vi "CCE MGLD PMJD PF SubVI05.vi"(6 "Coordenadas":T2, 8 "DireccionMemoria":path, 9 "UMBRAL":u8(knob) scale=0.0..255.0, 10 "Tolerancia":dbl, 11 "Image":T1) -> (0 "Estado botella":string, 2 "Abolladuas?":bool)   [LabVIEW 2020]
uses:
  <vilib>/vision/Image Controls.llb/IMAQ Image.ctl
panel:
  out "Image 2":T1(plugin-control)
  out "Diferencia":dbl
  out "Memoria":picture
  out "Muestra":picture
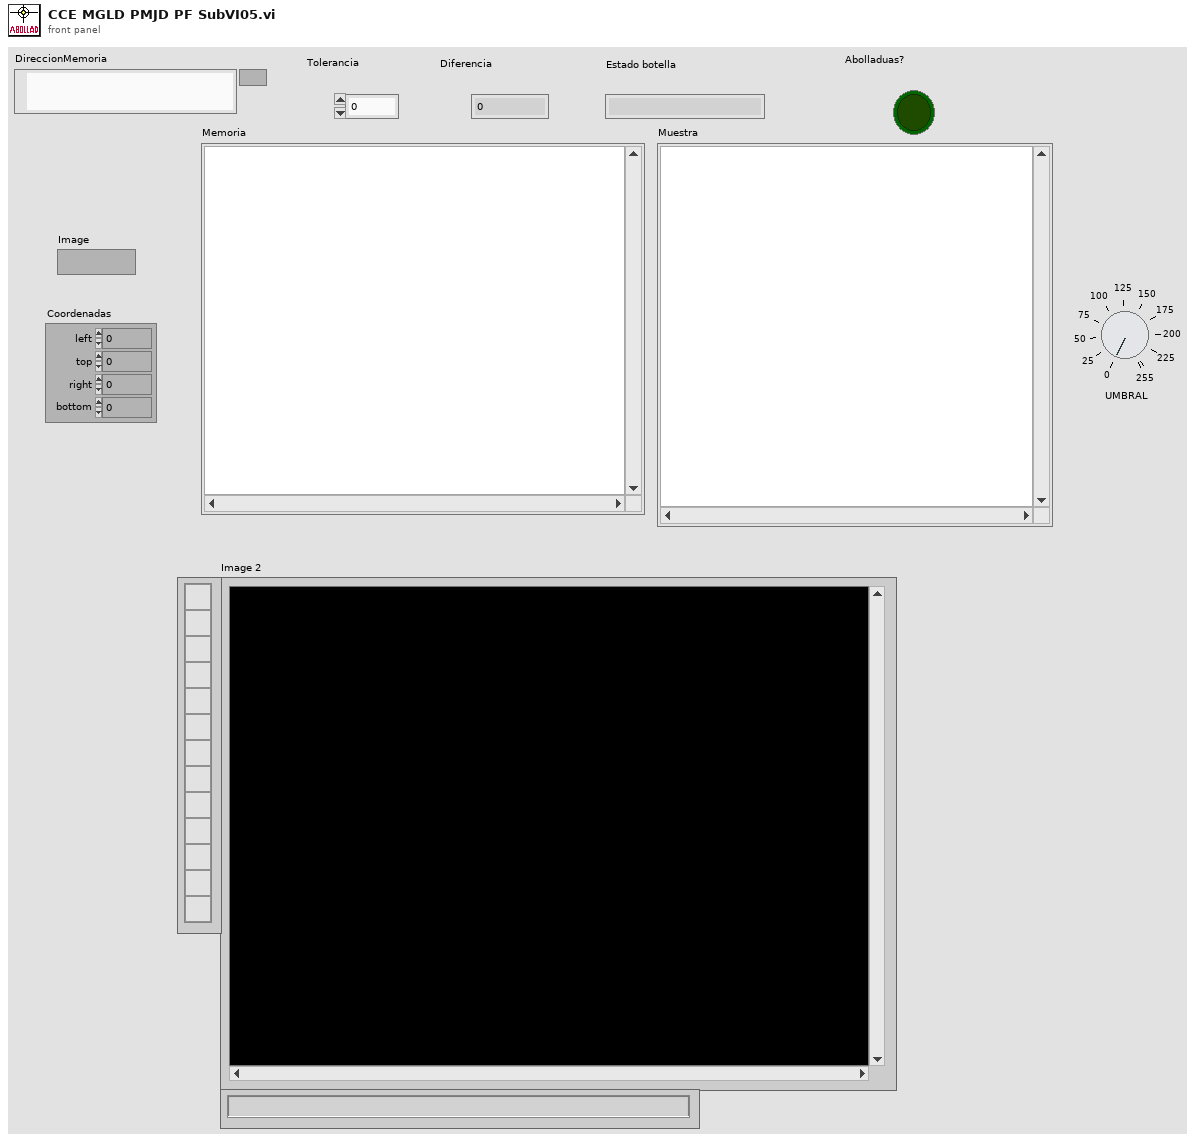
[diagram p1: front panel]
types:
  T1 = typedef "IMAQ Image.ctl" = refnum<image>
  T2 = cluster{"left":i16, "top":i16, "right":i16, "bottom":i16}
  T3 = typedef "Image Type" = u32
  T4 = typedef "imagedata.ctl" = cluster{"image type":i32, "image depth":i32, "image":u8[], "mask":u8[], "colors":u32[], "Rectangle":cluster{"left":i16, "top":i16, "right":i16, "bottom":i16}}
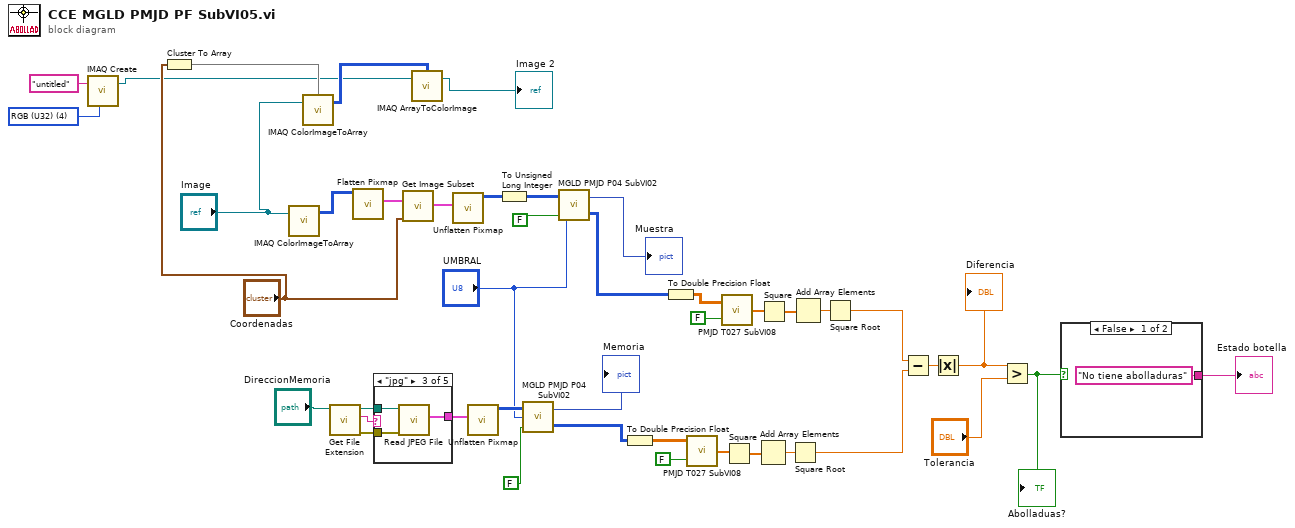
[diagram p0: block diagram]
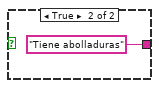
[diagram p2: hidden frame]
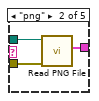
[diagram p4: hidden frame]
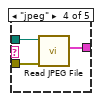
[diagram p5: hidden frame]
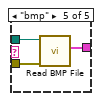
[diagram p6: hidden frame]
diagram:
  w1 = T3 4 items=["Grayscale (U8)", "Grayscale (I16)", "Grayscale (SGL)", "Complex (CSG)", "RGB (U32)", "HSL (U32)", "RGB (U64)", "Grayscale (U16)"] ("Image Type")
  n1 = call "IMAQ Create"("Image Name"="untitled", "Image Type"=w1) -> ("New Image"=w3:T1)  [unwired: 3 in, 1 out]
  n2 = Cluster To Array(cluster="Coordenadas") -> (array=w5:i16[])
  n3 = call "IMAQ ColorImageToArray"("Image"="Image") -> ("Image Pixels (U32)"=w10:u32[][])  [unwired: 3 in, 2 out]
  n4 = call "IMAQ ColorImageToArray"("Optional Rectangle"=w5, "Image"="Image") -> ("Image Pixels (U32)"=w7:u32[][])  [unwired: 2 in, 2 out]
  n5 = call <vilib>:"Get File Extension.vi"("file"="DireccionMemoria") -> ("error out"=w39:errorcluster, "lowercase file extension"=w41:string, "dup file"=w40:path)  [unwired: 6 in, 2 out]
  n6 = call <vilib>:"Flatten Pixmap.vi"("24-bit pixmap"=w10) -> ("image data"=w13:T4)  [unwired: 10 in]
  n7 = case shown="\"jpg\"" w41 {
    tunnel: w40 -> [_ w46 w47 w52 w54]
    tunnel: w39 -> [_ w45 w49 w51 w55]
    tunnel: [_ w44 w48 w50 w53] -> w38
    frame "False", Default {
    }
    frame "png" {
      n8 = call <vilib>:"Read PNG File.vi"("error in (no error)"=w45, "path to PNG file"=w46) -> ("image data"=w44:T4)  [unwired: 7 in, 2 out]
    }
    frame "jpg" {
      n9 = call <vilib>:"Read JPEG File.vi"("error in (no error)"=w49, "path to JPEG file"=w47) -> ("image data"=w48:T4)  [unwired: 7 in, 2 out]
    }
    frame "jpeg" {
      n10 = call <vilib>:"Read JPEG File.vi"("error in (no error)"=w51, "path to JPEG file"=w52) -> ("image data"=w50:T4)  [unwired: 7 in, 2 out]
    }
    frame "bmp" {
      n11 = call <vilib>:"Read BMP File.vi"("error in (no error)"=w55, "path to BMP file"=w54) -> ("image data"=w53:T4)  [unwired: 7 in, 2 out]
    }
  }
  n12 = call <vilib>:"Get Image Subset.vi"("subset rect"="Coordenadas", "image data"=w13) -> ("image subset"=w12:T4)  [unwired: 4 in, 1 out]
  n13 = call "IMAQ ArrayToColorImage"("Image Pixels (U32)"=w7, "Image"=w3) -> ("Image Out"=→"Image 2":T1)  [unwired: 3 in, 1 out]
  n14 = call <vilib>:"Unflatten Pixmap.vi"("image data"=w12) -> ("24-bit pixmap"=w11:u32[][])  [unwired: 4 in, 6 out]
  n15 = call <vilib>:"Unflatten Pixmap.vi"("image data"=w38) -> ("24-bit pixmap"=w36:u32[][])  [unwired: 4 in, 6 out]
  n16 = To Unsigned Long Integer(number=w11) -> (unsigned 32bit integer=w14:u32[][])
  n17 = call "MGLD PMJD P04 SubVI02.vi"("INVERTIDO?"=FALSE, "UMBRAL"="UMBRAL", "pixmap"=w36) -> ("Umbralizado"=w16:u8[][], "IMG"=→"Memoria":picture)
  n18 = call "MGLD PMJD P04 SubVI02.vi"("INVERTIDO?"=FALSE, "UMBRAL"="UMBRAL", "pixmap"=w14) -> ("Umbralizado"=w18:u8[][], "IMG"=→"Muestra":picture)
  n19 = To Double Precision Float(number=w16) -> (double precision float=w17:dbl[][])
  n20 = To Double Precision Float(number=w18) -> (double precision float=w19:dbl[][])
  n21 = call "PMJD T027 SubVI08.vi"("NORMALIZACIÓN"=FALSE, "f"=w17) -> ("MOMENTOS Hu"=w34:dbl[])
  n22 = call "PMJD T027 SubVI08.vi"("NORMALIZACIÓN"=FALSE, "f"=w19) -> ("MOMENTOS Hu"=w29:dbl[])
  n23 = Square(x=w34) -> (x^2=w33:dbl[])
  n24 = Add Array Elements(numeric array=w33) -> (sum=w32:dbl)
  n25 = Square(x=w29) -> (x^2=w31:dbl[])
  n26 = Square Root(x=w32) -> (sqrt(x)=w27:dbl)
  n27 = Add Array Elements(numeric array=w31) -> (sum=w30:dbl)
  n28 = Square Root(x=w30) -> (sqrt(x)=w28:dbl)
  n29 = Subtract(x=w28, y=w27) -> (x-y=w26:dbl)
  n30 = Absolute Value(x=w26) -> (abs(x)=w25:dbl)
  "Diferencia" <- w25
  n31 = Greater?(x=w25, y="Tolerancia") -> (0:w24:bool)
  "Abolladuas?" <- w24
  n32 = case shown="False" w24 {
    tunnel: ["No tiene abolladuras" "Tiene abolladuras"] -> w23
    frame False {
    }
    frame True {
    }
  }
  "Estado botella" <- w23
